vi "OCR-车牌识别2.vi"(0 "ROI Descriptor (OCR/OCV 1)":T2={"Global Rectangle"=[455, 94, 585, 233], "Contours"=[{"ID"=enum."External", "Type"=3, "Coordinates"=[455, 94, 585, 233]}]} {"Contours"."Type" items=["No Selection", "Point", "Line", "Rectangle", "Oval", "Polygon", "Freehand Region", "Annulus", "Unused2", "Unused3", "Broken Line", "Freehand Line", "Rotated Rectangle"]}, 1 "File Path (OCR/OCV 1)":path=path "D:/Labviewprogram/视觉/视觉框架/NEW-车牌号.abc", 2 "Parameters (OCR/OCV 1)":T1={"Threshold Data"={"Method"=enum."Uniform", "Looking for"=1, "Color Mode"=0, "Kernel Size"={"Width"=32, "Height"=32}, "Ranges"=[{"Min"=1, "Max"=255}]}, "Reject Border"=TRUE, "Number Of Erosions"=0, "Size & Spacing"={"Segment Algorithm"=0, "Min Bounding Rect Width"=1, "Max Bounding Rect Width"=65536, "Min Bounding Rect Height"=1, "Max Bounding Rect Height"=65536, "Min Character Size"=20, "Max Character Size"=65536, "Min Char Spacing"=1, "Max Horiz Element Spacing"=1, "Max Vert Element Spacing"=0, "Max Space Distance"=65536}, "Read Options"={"Read Strategy"=1, "Read Resolution"=2, "Scale Dependant"=FALSE, "Aspect Ratio"=400, "Acceptance Level"=700, "Substitution Character"="?", "MultiLine"=TRUE}, "Valid Characters"=[], "Use Text Pattern"=FALSE, "Orientation"=0, "# Lines Expected"=0, "Number of Blocks"=4} {"Threshold Data"."Looking for" items=["Light on Dark", "Dark on Light"]; "Threshold Data"."Color Mode" items=["RGB", "HSL", "HSV", "HSI"]; "Size & Spacing"."Segment Algorithm" items=["None", "Shortest Segment", "Legacy Auto Split"]; "Read Options"."Read Strategy" items=["Aggressive", "Conservative"]; "Read Options"."Read Resolution" items=["Low", "Medium", "High"]; "Valid Characters"."Pre-defined characters" items=["Any Character", "User-defined Characters", "Alphabetic", "Alphanumeric", "Uppercase Letters", "Lowercase Letters", "Decimal Digits", "Hexadecimal Digits", "Pattern", "Force Space"]; "Orientation" items=["Baseline inside", "Baseline outside"]}, 7 "error in":errorcluster) -> (20 "String (OCR/OCV 1)":string, 21 "OCR Session (OCR/OCV 1)":T4, 27 "error out":errorcluster)   [LabVIEW 2018]
uses:
  <vilib>/vision/OCR.llb/IMAQ OCR Session.ctl
  <vilib>/vision/NI_Vision_Development_Module.lvlib
panel:
  out "Image Out":T3(plugin-control)
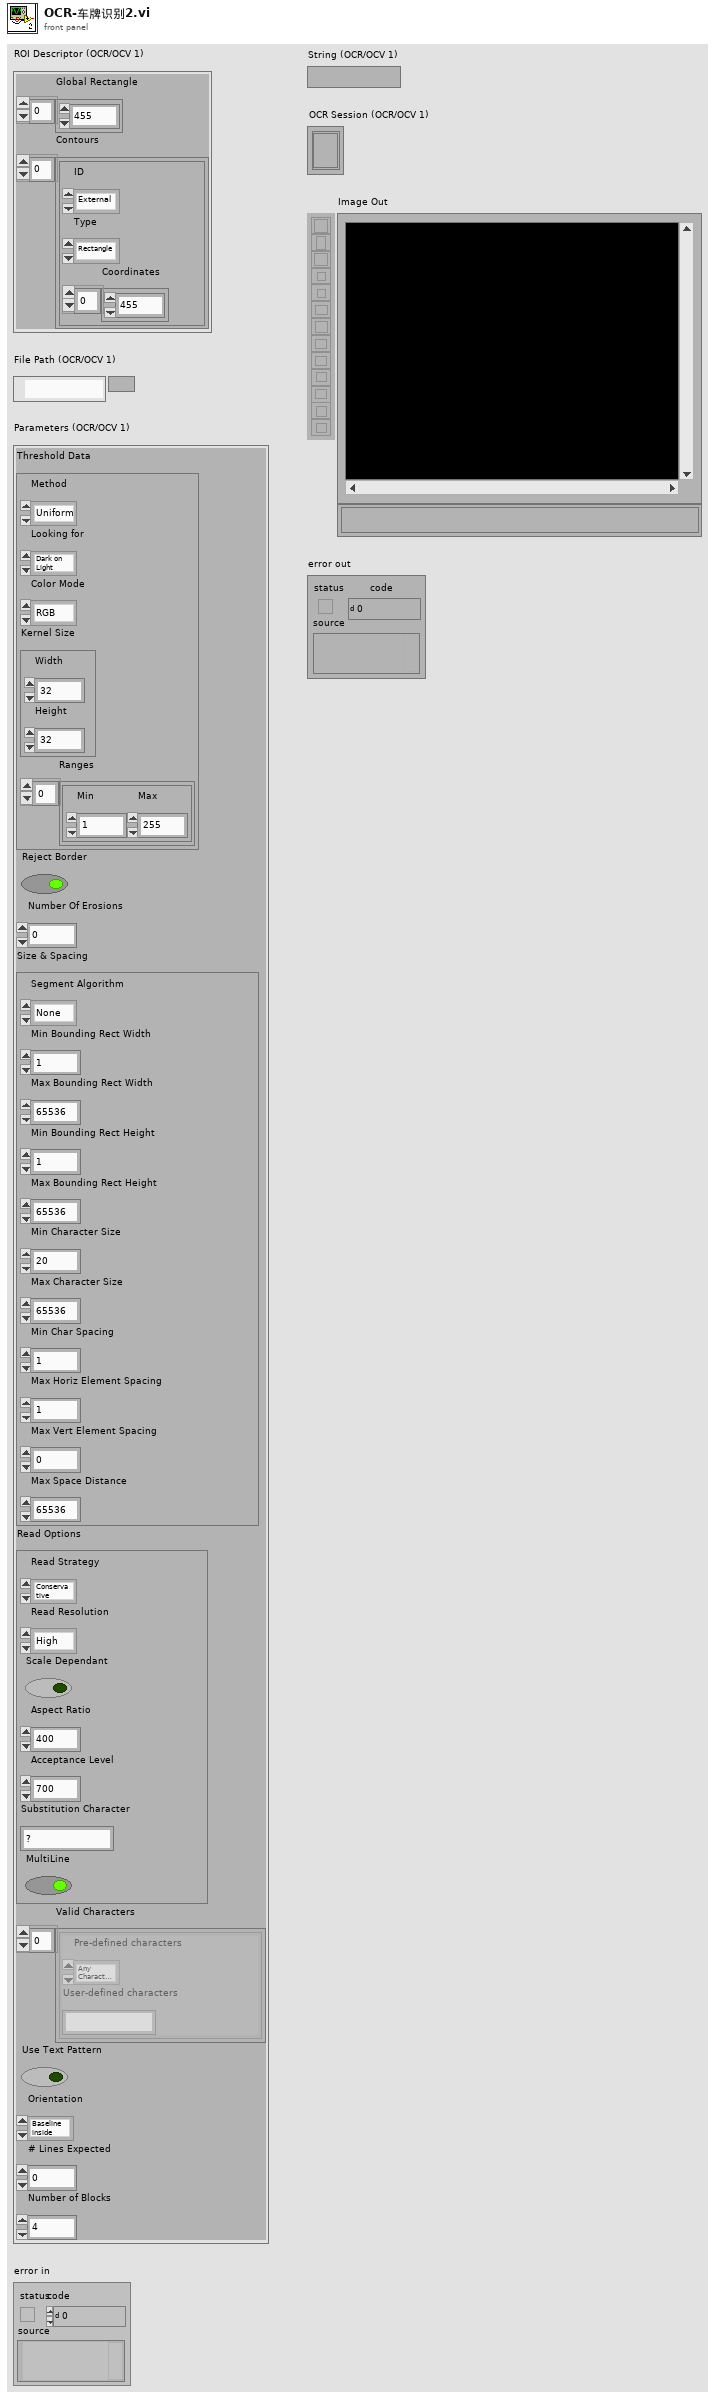
[diagram p1: front panel]
types:
  T1 = cluster{"Threshold Data":cluster{"Method":enum16{"Fixed Range", "Uniform", "Linear", "Non Linear", "Local", "Color"}, "Looking for":u32, "Color Mode":u32, "Kernel Size":cluster{"Width":i32, "Height":i32}, "Ranges":cluster{"Min":i32, "Max":i32}[]}, "Reject Border":bool, "Number Of Erosions":i32, "Size & Spacing":cluster{"Segment Algorithm":u16, "Min Bounding Rect Width":i32, "Max Bounding Rect Width":i32, "Min Bounding Rect Height":i32, "Max Bounding Rect Height":i32, "Min Character Size":i32, "Max Character Size":i32, "Min Char Spacing":i32, "Max Horiz Element Spacing":i32, "Max Vert Element Spacing":i32, "Max Space Distance":i32}, "Read Options":cluster{"Read Strategy":i32, "Read Resolution":i32, "Scale Dependant":bool, "Aspect Ratio":i32, "Acceptance Level":i32, "Substitution Character":string, "MultiLine":bool}, "Valid Characters":cluster{"Pre-defined characters":i32, "User-defined characters":string}[], "Use Text Pattern":bool, "Orientation":u32, "# Lines Expected":u32, "Number of Blocks":i32}
  T2 = cluster{"Global Rectangle":i32[], "Contours":cluster{"ID":enum32{"External", "Internal"}, "Type":u32, "Coordinates":i32[]}[]}
  T3 = typedef "IMAQ Image.ctl" = refnum<image>
  T4 = typedef "IMAQ OCR Session.ctl" = refnum<k1>
  T5 = typedef "Image Type" = u32
  T6 = cluster{"Global Rectangle":i32[], "Contours":cluster{"Contour Type":u32, "ROI Type":u32, "Points":i32[]}[]}
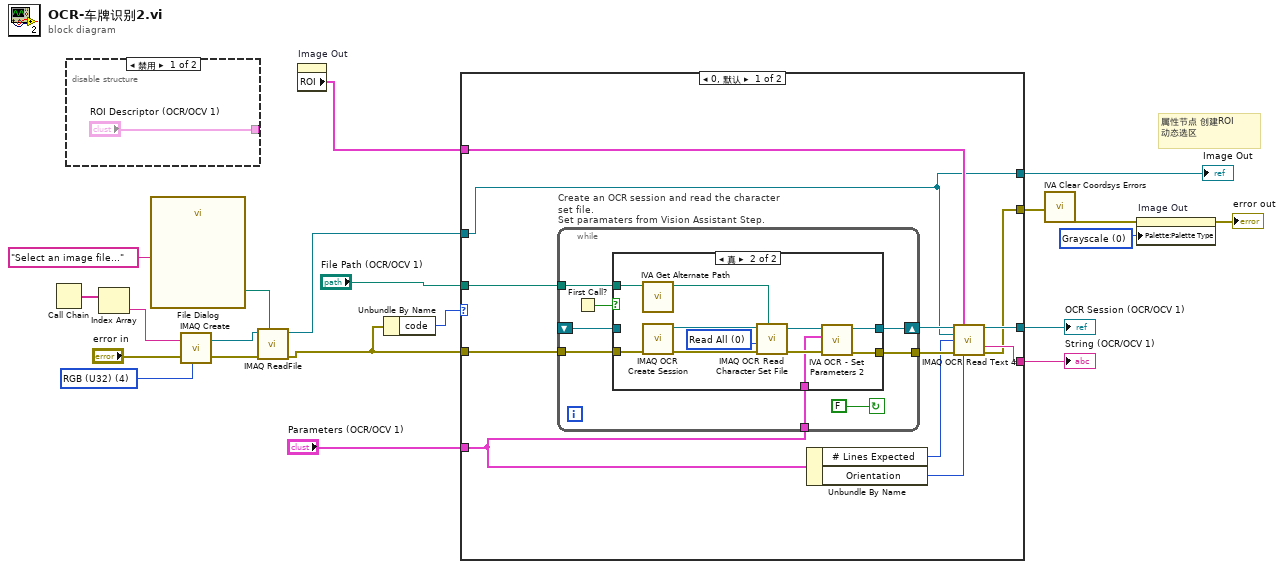
[diagram p0: block diagram]
diagram:
  w5 = u32 0 items=["Grayscale", "Binary", "Gradient", "Rainbow", "Temperature", "User Defined", "Binary 16 Bit", "Gradient 16 Bit", "Rainbow 16 Bit", "Temperature 16 Bit", "User Defined 16 Bit"] ("Palette Type")
  w14 = T5 4 items=["Grayscale (U8)", "Grayscale (I16)", "Grayscale (SGL)", "Complex (CSG)", "RGB (U32)", "HSL (U32)", "RGB (U64)", "Grayscale (U16)"] ("Image Type")
  # "属性节点 创建ROI\n动态选区"
  n1 = Call Chain() -> (call chain=w18:string[])
  n2 = disable-structure shown="禁用" {
    disable-tunnel: ["ROI Descriptor (OCR/OCV 1)" _] -> _
    frame Disabled {
    }
    frame Enabled {
    }
  }
  n3 = Index Array(array=w18) -> (element=w17:string)  [unwired: 1 in]
  n4 = call "File Dialog"("prompt"="Select an image file...") -> ("selected path"=w15:path)  [unwired: 6 in, 8 out]
  n5 = call "IMAQ Create"("Image Name"=w17, "Image Type"=w14, "error in (no error)"="error in") -> ("New Image"=w21:T3, "error out"=w20:errorcluster)  [unwired: 1 in, 1 out]
  n6 = call "IMAQ ReadFile"("File Path"=w15, "error in (no error)"=w20, "Image"=w21) -> ("error out"=w4:errorcluster, "Image Out"=w6:T3)  [unwired: 2 in, 5 out]
  n7 = property on="Image Out" class="ImageControl"() -> ("ROI"=w1:T6)  [unwired: 2 in, 2 out]
  n8 = Unbundle By Name(w4) -> ("code"=w3:i32)
  n9 = case shown="0, 默认" w3 {
    tunnel: w4 -> [w34 _]
    tunnel: "File Path (OCR/OCV 1)" -> [w33 _]
    tunnel: [w32 _] -> w12
    tunnel: w1 -> [w31 _]
    tunnel: [w30 _] -> w11
    tunnel: "Parameters (OCR/OCV 1)" -> [w29 _]
    tunnel: [w24 _] -> w9
    tunnel: w6 -> [w23 _]
    tunnel: [w23 _] -> w2
    frame 0, Default {
      n10 = while "Create an OCR session and read the character set file.\nSet paramaters from Vision Assistant Step." {
        shift-right: [w39] -> w27
        shift-left: _ -> [w38]
        tunnel: w34 -> [w41]
        tunnel: w29 -> [w37]
        tunnel: w33 -> [w36]
        tunnel: [w35] -> w28
        stop <- FALSE continue-if-true
        n11 = First Call?() -> (First Call?: T/F=w40:bool)
        n12 = case "条件结构" shown="真" w40 {
          tunnel: w36 -> [_ w48]
          tunnel: w41 -> [w43 w52]
          tunnel: [w44 w50] -> w39
          tunnel: [w43 w49] -> w35
          tunnel: w37 -> [_ w45]
          tunnel: w38 -> [w44 _]
          frame False {
          }
          frame True {
            w53 = 0 items=["Read All", "Read Character Set Only", "Read Properties Only"] ("Read Options")
            n13 = call <vilib>:"IVA Get Alternate Path.vi"("Path In"=w48) -> ("Path Out"=w47:path)  [unwired: 10 out]
            n14 = call "IMAQ OCR Create Session"("error in (no error)"=w52) -> ("error out"=w54:errorcluster, "IMAQ OCR Session"=w55:T4)  [unwired: 9 out]
            n15 = call "IMAQ OCR Read Character Set File"("File Path"=w47, "error in (no error)"=w54, "Read Options"=w53, "IMAQ OCR Session"=w55) -> ("error out"=w51:errorcluster, "IMAQ OCR Session (dup)"=w46:T4)  [unwired: 1 in, 5 out]
            n16 = call <vilib>:"IVA OCR - Set Parameters 2.vi"("error in (no error)"=w51, "Parameters"=w45, "IMAQ OCR Session"=w46) -> ("error out"=w49:errorcluster, "IMAQ OCR Session Out"=w50:T4)  [unwired: 7 in]
          }
        }
      }
      n17 = Unbundle By Name(w29) -> ("# Lines Expected"=w25:u32, "Orientation"=w26:u32)
      n18 = call "IMAQ OCR Read Text 4"("IMAQ OCR Session"=w27, "ROI Descriptor"=w31, "Image"=w23, "Number of Lines Requested"=w25, "error in (no error)"=w28, "Orientation"=w26) -> ("IMAQ OCR Session (dup)"=w30:T4, "Read String"=w32:string, "error out"=w24:errorcluster)  [unwired: 7 out]
    }
    frame 1 {
    }
  }
  "String (OCR/OCV 1)" <- w12
  "OCR Session (OCR/OCV 1)" <- w11
  "Image Out" <- w2
  n19 = call <vilib>:"IVA Clear Coordsys Errors.vi"("error in (no error)"=w9) -> ("error out"=w8:errorcluster)  [unwired: 10 in]
  n20 = property on="Image Out" class="ImageControl"(error in=w8, "Palette:Palette Type"=w5) -> (error out=→"error out":errorcluster)  [unwired: 1 in, 1 out]
